vi "Get JSON Param Documentation (default).vi"(8 "error in (no error)":errorcluster, 10 "request cluster":variant) -> (0 "error out":errorcluster, 2 "<JSON> Request Documentation":string)   [LabVIEW 2019, in "Help.lvclass"]
uses:
  Help.lvclass
  46988592-c207-47b7-8b61-3fcb2b203627.vi
  <vilib>/JDP Science/JSONtext/Variant to JSON Text.vi
  <vilib>/JDP Science/JSONtext/LVClass Serializer/JSONtext LVClass Serializer.lvclass
  <vilib>/JDP Science/JSONtext/JSONtext.lvlib
  <vilib>/Utility/Data Type/NI_Data Type.lvlib
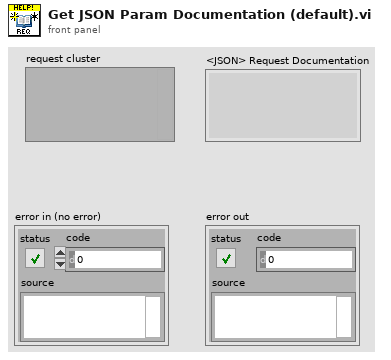
[diagram p1: front panel]
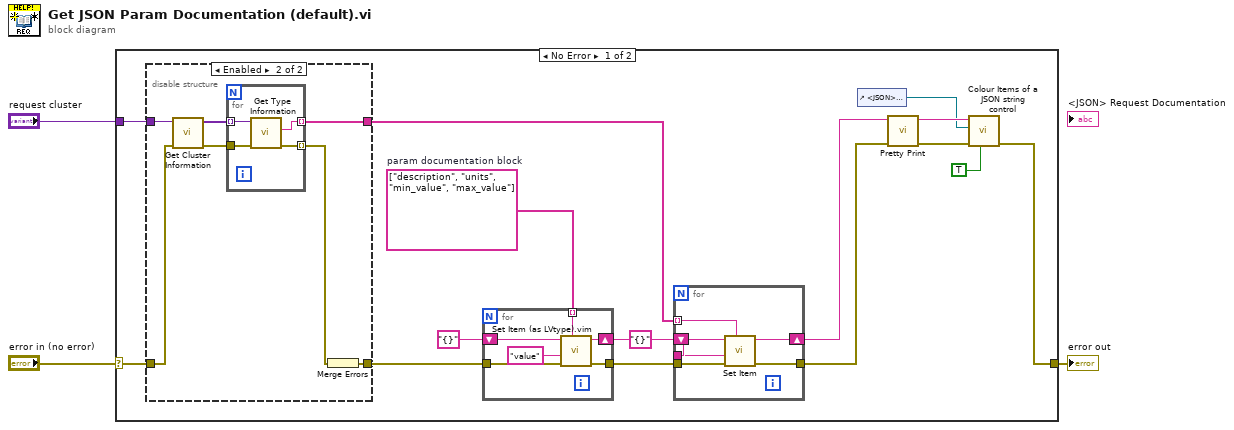
[diagram p0: block diagram]
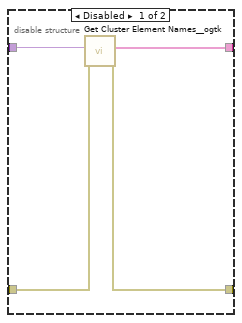
[diagram p2: hidden frame]
diagram:
  n1 = case shown="No Error" "error in (no error)" {
    selector: "error in (no error)" -> [w11 w47]
    tunnel: "request cluster" -> [w19 _]
    tunnel: [w4 w47] -> w1
    frame No Error {
      w13 = string[] ["description", "units", "min_value", "max_value"]  # param documentation block
      n2 = disable-structure shown="Enabled" {
        disable-tunnel: w19 -> [w23 w30]
        disable-tunnel: [w22 w28] -> w15
        disable-tunnel: [w21 w24] -> w12
        disable-tunnel: w11 -> [w20 w26]
        frame Disabled {
          n3 = call <userlib>:"Get Cluster Element Names__ogtk.vi"("error in (no error)"=w20, "Cluster"=w23) -> ("error out"=w21:errorcluster, "Element Names"=w22:string[])  [unwired: 8 in]
        }
        frame Enabled {
          n4 = call <vilib>:"Get Cluster Information.vi"("error in (no error)"=w26, "variant"=w30) -> ("error out"=w27:errorcluster, "cluster elements"=w29:variant[])  [unwired: 8 in]
          n5 = for {
            tunnel: w29 -> [w34] mode=indexing
            tunnel: [w33] -> w28 mode=indexing
            tunnel: w27 -> [w32]
            tunnel: [w31] -> w25 mode=indexing
            n6 = call <vilib>:"Get Type Information.vi"("error in (no error)"=w32, "variant"=w34) -> ("error out"=w31:errorcluster, "name"=w33:string)  [unwired: 5 in, 3 out]
          }
          n7 = Merge Errors(w25) -> (w24:errorcluster)
        }
      }
      n8 = for {
        tunnel: w13 -> [w45] mode=indexing
        shift-right: [w44] -> w17
        shift-left: "{}" ("JSON") -> [w46]
        tunnel: [w43] -> w16
        tunnel: w12 -> [w41]
        n9 = call "Set Item (as LVtype).vim"("$Path or Item Name"=w45, "error in (no error)"=w41, "Anything"="value", "JSON"=w46) -> ("error out"=w43:errorcluster, "<JSON>"=w44:string)  [unwired: 4 in, 1 out]
      }
      n10 = for {
        shift-right: [w39] -> w7
        shift-left: "{}" ("JSON") -> [w40]
        tunnel: [w38] -> w5
        tunnel: w17 -> [w37]
        tunnel: w15 -> [w36] mode=indexing
        tunnel: w16 -> [w35]
        n11 = call <vilib>:"Set Item.vi"("$Path or Item Name"=w36, "error in (no error)"=w35, "JSON to Insert"=w37, "JSON"=w40) -> ("error out"=w38:errorcluster, "<JSON>"=w39:string)  [unwired: 4 in, 1 out]
      }
      n12 = control-ref of="<JSON> Request Documentation"() -> (w6:refnum<vi>)
      n13 = call <vilib>:"Pretty Print.vi"("error in (no error)"=w5, "JSON"=w7) -> ("error out"=w9:errorcluster, "<JSON>"=w8:string)  [unwired: 7 in, 1 out]
      n14 = call <vilib>:"Colour Items of a JSON string control.vi"("Defer Panel Updates"=TRUE, "error in (no error)"=w9, "String Control"=w6, "JSON"=w8) -> ("error out"=w4:errorcluster)  [unwired: 7 in]
    }
    frame Error {
    }
  }
  "error out" <- w1
